vi "Home.vi"(8 "error in (no error)":errorcluster, 10 "VISA resource name in":refnum<visa-resource-name>, 11 "LCD-I2C in":refnum<class "LCD-I2C.lvclass">) -> (0 "error out":errorcluster, 2 "VISA resource name":refnum<visa-resource-name>, 3 "LCD-I2C out":refnum<class "LCD-I2C.lvclass">)   [LabVIEW 2023, in "CTI-Visa-DeviceLib.lvlib" / "LCD-I2C.lvclass"]
uses:
  LCD-I2C.lvclass
  Command.ctl
  cf145065-4270-436c-bc9a-ee197729c93e.vi
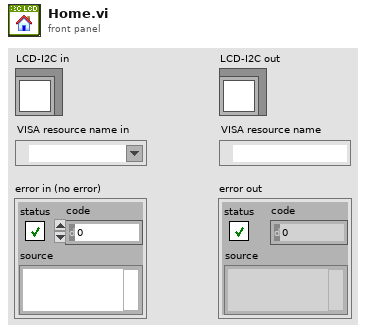
[diagram p1: front panel]
types:
  T1 = typedef "CTI-Visa-DeviceLib.lvlib/LCD-I2C.lvclass/Command.ctl" = enum16{"Clear Display", "Return Home", "Entry Mode Set", "Display Control", "Cursor Shift", "Function Set", "Set CGRAM Addr", "Set DDRAM Addr"}
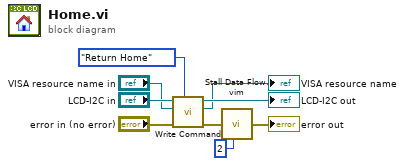
[diagram p0: block diagram]
diagram:
  n1 = call "Write Command.vi"("Command"=Command."Return Home", "error in (no error)"="error in (no error)", "VISA resource name in"="VISA resource name in", "LCD-I2C in"="LCD-I2C in") -> ("error out"=w8:errorcluster, "VISA resource name"=→"VISA resource name":refnum<visa-resource-name>, "LCD-I2C out"=→"LCD-I2C out":refnum<class "LCD-I2C.lvclass">)  [unwired: 5 in]
  n2 = call "Stall Data Flow.vim"("value in"=w8, "milliseconds to wait"=u32 2) -> ("value out"=→"error out":errorcluster)  [unwired: 1 out]
